vi "Loader.vi"(9 "Loader Name":string, 10 "PID":u32) -> ()   [LabVIEW 2021, in "PluginLoader.lvlib"]
uses:
  PluginLoader.lvlib
  CIFPluginLoader/CIFPluginLoader.lvclass
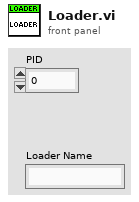
[diagram p1: front panel]
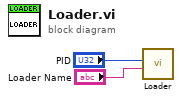
[diagram p0: block diagram]
diagram:
  n1 = call "Loader.vi"("Loader Name"="Loader Name", "PID"="PID") -> ()  [unwired: 10 in]
